vi "IMAQ Stack to Pointers.vi"(8 "error in":errorcluster, 10 "Number of threads":i32, 11 "IMAQ Image Array":T1[](array[typedef])) -> (0 "error out":errorcluster, 3 "Pointers Out":u64[](array[numeric]))   [LabVIEW 2013, in "KLB.lvlib"]
doc: "IMAQ Image Stack to Pointers.\n\nUses LabVIEW memory manager functions to quickly convert a stack of images into 1D arrays. The result is given as pointers to the 1D arrays.\n\nWill not function correctly for single images larger then 4GB.\n\nWill correctly remove any whitespace from IMAQ images.\n\nFree pointers with \nLibrary - LabVIEW \nFunction - DSDisposePtr\nwhen done with pointers"
uses:
  KLB.lvlib
  <vilib>/vision/Image Controls.llb/IMAQ Image.ctl
panel:
  # "Free pointers with\nLabVIEW\nDSDisposePtr\n\nSee LabVIEW help - memory manger for\nmore information"
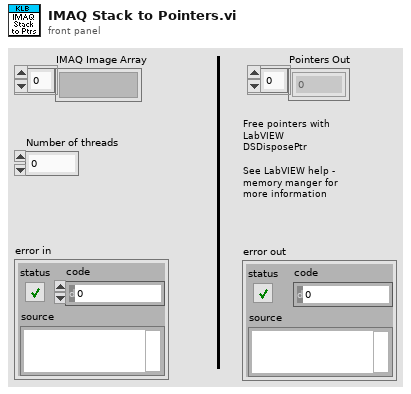
[diagram p1: front panel]
types:
  T1 = typedef "IMAQ Image.ctl" = refnum<image>
  T2 = enum32{"Map Pixel Pointer", "Unmap Pixel Pointer", "Get Pixels Infos"}
  T3 = typedef "Image Type" = u32
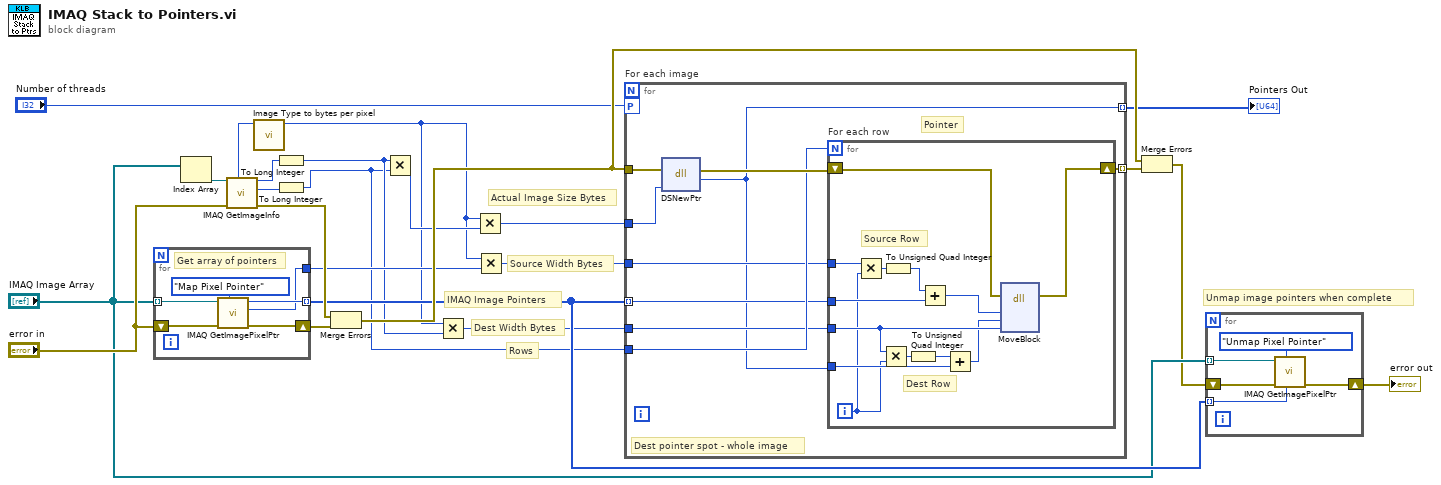
[diagram p0: block diagram]
diagram:
  # "Unmap image pointers when complete"
  # "Rows"
  # "Dest Width Bytes"
  # "Source Width Bytes"
  # "Actual Image Size Bytes"
  # "IMAQ Image Pointers"
  n1 = for {
    tunnel: "IMAQ Image Array" -> [w25] mode=indexing
    tunnel: [w28] -> w20 mode=indexing
    shift-right: [w26] -> w1
    shift-left: "error in" -> [w27]
    tunnel: [w24] -> w9
    # "Get array of pointers"
    n2 = call "IMAQ GetImagePixelPtr"("Function"=T2."Map Pixel Pointer", "error in (no error)"=w27, "Image"=w25) -> ("error out"=w26:errorcluster, "LineWidth(Pixels)"=w24:i32, "Pixel Pointer out"=w28:u64)  [unwired: 3 in, 3 out]
  }
  n3 = Index Array(array="IMAQ Image Array") -> (element=w17:T1)  [unwired: 1 in]
  n4 = call "IMAQ GetImageInfo"("error in (no error)"="error in", "Image"=w17) -> ("error out"=w22:errorcluster, "Y Resolution"=w15:i32, "X Resolution"=w16:i32, "Image Type"=w14:T3)  [unwired: 2 in, 4 out]
  n5 = call "Image Type to bytes per pixel.vi"("Image Type"=w14) -> ("Bytes per Pixel"=w2:u32)  [unwired: 10 in]
  n6 = To Long Integer(number=w16) -> (32bit integer=w4:i32)
  n7 = To Long Integer(number=w15) -> (32bit integer=w3:i32)
  n8 = Merge Errors(w22, w1) -> (w21:errorcluster)
  n9 = Multiply(x=w4, y=w3) -> (x*y=w13:i32)
  n10 = Multiply(x=w2, y=w4) -> (x*y=w11:u32)
  n11 = Multiply(x=w2, y=w13) -> (x*y=w12:u32)
  n12 = Multiply(x=w2, y=w9) -> (x*y=w10:u32)
  n13 = for "For each image" {
    tunnel: w20 -> [w35] mode=indexing
    tunnel: w12 -> [w31]
    workers-P: "Number of threads" -> [_]
    tunnel: w10 -> [w34]
    tunnel: w11 -> [w36]
    tunnel: w3 -> [w37]
    tunnel: w21 -> [w32]
    tunnel: [w33] -> w8 mode=indexing
    tunnel: [w30] -> w5 mode=indexing
    # "Pointer"
    # "Dest pointer spot - whole image"
    n14 = dll-call lib="LabVIEW" fn="DSNewPtr"(error in=w32, "Size"=w31) -> (error out=w38:errorcluster, "Pointer"=w30:u64)  [unwired: 3 in, 1 out]
    n15 = for "For each row" {
      N: w37 -> [_]
      tunnel: w36 -> [w43]
      tunnel: w35 -> [w50]
      tunnel: w34 -> [w49]
      tunnel: w30 -> [w51]
      shift-right: [w39] -> w33
      shift-left: w38 -> [w40]
      i -> [w42]
      # "Dest Row"
      # "Source Row"
      n16 = Multiply(x=w49, y=w42) -> (x*y=w46:u32)
      n17 = Multiply(x=w43, y=w42) -> (x*y=w44:u32)
      n18 = To Unsigned Quad Integer(1:w46) -> (0:w47:u64)
      n19 = To Unsigned Quad Integer(1:w44) -> (0:w45:u64)
      n20 = Add(x=w47, y=w50) -> (x+y=w48:u64)
      n21 = Add(x=w45, y=w51) -> (x+y=w41:u64)
      n22 = dll-call lib="LabVIEW" fn="MoveBlock"(error in=w40, "Source"=w48, "Destination"=w41, "Size"=w43) -> (error out=w39:errorcluster)  [unwired: 6 in, 1 out]
    }
  }
  "Pointers Out" <- w5
  n23 = Merge Errors(w21, w8) -> (w18:errorcluster)
  n24 = for {
    shift-right: [w54] -> w6
    shift-left: w18 -> [w55]
    tunnel: "IMAQ Image Array" -> [w53] mode=indexing
    tunnel: w20 -> [w52] mode=indexing
    n25 = call "IMAQ GetImagePixelPtr"("Pixel Pointer in"=w52, "Function"=T2."Unmap Pixel Pointer", "error in (no error)"=w55, "Image"=w53) -> ("error out"=w54:errorcluster)  [unwired: 2 in, 5 out]
  }
  "error out" <- w6
